vi "SubVI_VPdistance_normalized.vi"(1 "Cost":dbl, 2 "Test Object":dbl[](array[numeric]), 3 "Basis Object":dbl[](array[numeric])) -> (0 "VP Distance (normalized)":dbl)   [LabVIEW 2018]
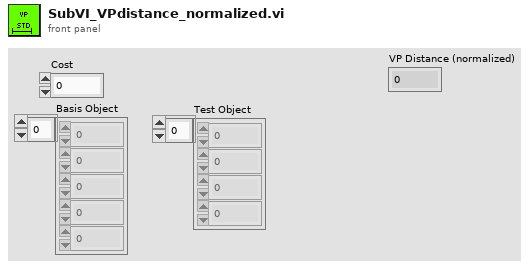
[diagram p1: front panel]
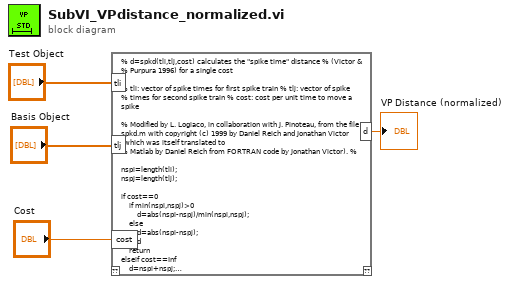
[diagram p0: block diagram]
diagram:
  n1 = script code="% d=spkd(tli,tlj,cost) calculates the \"spike time\" distance % (Victor &\n% Purpura 1996) for a single cost\n\n% tli: vector of spike times for first spike train % tlj: vector of spike\n% times for second spike train % cost: cost per unit time to move a spike\n\n% Modified by L. Logiaco, in collaboration with J. Pinoteau, from the file spkd.m with copyright (c) 1999 by Daniel Reich and Jonathan Victor (which was itself translated to\n% Matlab by Daniel Reich from FORTRAN code by Jonathan Victor). % \n\nnspi=length(tli);\nnspj=length(tlj);\n\nif cost==0\n    if min(nspi,nspj)>0\n        d=abs(nspi-nspj)/min(nspi,nspj);\n    else\n        d=abs(nspi-nspj);\n    end\n    return \nelseif cost==Inf\n    d=nspi+nspj; \n    return \nend \n\n\nscr=zeros(nspi+1,nspj+1);\n\n% % INITIALIZE MARGINS WITH COST OF ADDING A SPIKE % \n\nscr(:,1)=(0:nspi)';\nscr(1,:)=(0:nspj); \n\nmat_trace_nber_matched=zeros(nspi+1,nspj+1);\n\nif nspi & nspj \n    for i=2:nspi+1 \n        for j=2:nspj+1 \n            [scr(i,j),ind_min]=min([scr(i-1,j)+1 scr(i,j-1)+1 scr(i-1,j-1)+cost*abs(tli(i-1)-tlj(j-1))]);\n            switch ind_min\n                case 1\n                    mat_trace_nber_matched(i,j)=mat_trace_nber_matched(i-1,j);\n                case 2\n                    mat_trace_nber_matched(i,j)=mat_trace_nber_matched(i,j-1);\n                case 3\n                    mat_trace_nber_matched(i,j)=mat_trace_nber_matched(i-1,j-1)+1;\n            end\n        end\n    end\nend\nd=scr(nspi+1,nspj+1)/max(1,mat_trace_nber_matched(nspi+1,nspj+1));"("tli"="Test Object", "tlj"="Basis Object", "cost"="Cost") -> ("d"=→"VP Distance (normalized)":dbl)  [unwired: 1 in, 1 out]
